vi "SubRotate.vi"(8 "error in (no error)":errorcluster, 10 "input cluster":T1 {"Start X" scale=0.0..1024.0; "End X" scale=0.0..1024.0}, 11 "AVI Path":path) -> (0 "error out":errorcluster)   [LabVIEW 2013]
uses:
  <vilib>/vision/NI_Vision_Development_Module.lvlib
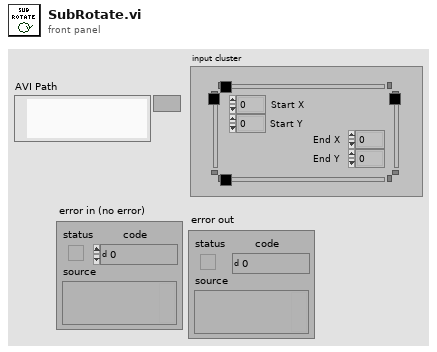
[diagram p1: front panel]
types:
  T1 = typedef "IMAQ Line" = cluster{"Start X":i32, "Start Y":i32, "End X":i32, "End Y":i32}
  T2 = cluster{cluster{i32, i32}, cluster{i32, i32}, cluster{"Start X":i32, "Start Y":i32}, cluster{"End X":i32, "End Y":i32}}
  T3 = typedef "AviRefnum.ctl" = refnum<k1>
  T4 = cluster{"width":u32, "height":u32, "framesPerSecond":u32, "compressionFilter":string, "hasData":bool}
  T5 = typedef "IMAQ Image.ctl" = refnum<image>
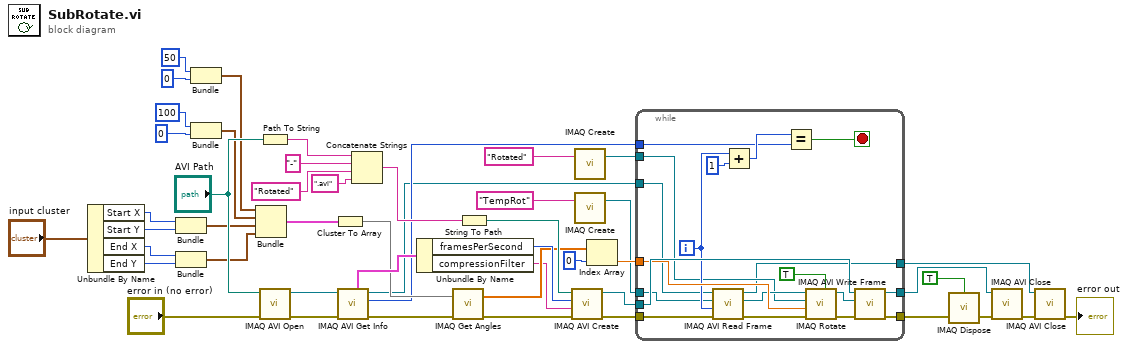
[diagram p0: block diagram]
diagram:
  n1 = Unbundle By Name("input cluster") -> ("Start X"=w30:i32, "Start Y"=w29:i32, "End X"=w28:i32, "End Y"=w27:i32)
  n2 = Bundle("Start X"=w30, "Start Y"=w29) -> (w26:cluster{"Start X":i32, "Start Y":i32})  [unwired: 1 in]
  n3 = Bundle("End X"=w28, "End Y"=w27) -> (w25:cluster{"End X":i32, "End Y":i32})  [unwired: 1 in]
  n4 = Bundle(50, 0) -> (w32:cluster{i32, i32})  [unwired: 1 in]
  n5 = Bundle(100, 0) -> (w31:cluster{i32, i32})  [unwired: 1 in]
  n6 = Bundle(w32, w31, w26, w25) -> (w24:T2)  [unwired: 1 in]
  n7 = Path To String(path="AVI Path") -> (string=w43:string)
  n8 = call "IMAQ AVI Open"("error in (no error)"="error in (no error)", "AVI Path"="AVI Path") -> ("error out"=w48:errorcluster, "Avi Refnum"=w47:T3)  [unwired: 8 in]
  n9 = Cluster To Array(cluster=w24) -> (array=w23:cluster{"End X":i32, "End Y":i32}[])
  n10 = call "IMAQ AVI Get Info"("error in (no error)"=w48, "Avi Refnum"=w47) -> ("error out"=w5:errorcluster, "Number of Frames"=w19:u32, "Avi Refnum (duplicate)"=w4:T3, "Frame Data"=w46:T4)  [unwired: 5 in, 1 out]
  n11 = Concatenate Strings(w43, "-" ("string"), "Rotated" ("string"), ".avi" ("string")) -> (w40:string)
  n12 = Unbundle By Name(w46) -> ("framesPerSecond"=w45:u32, "compressionFilter"=w18:string)
  n13 = call "IMAQ Get Angles"("error in (no error)"=w5, "Points"=w23) -> ("error out"=w17:errorcluster, "Angles (deg)"=w22:sgl[])  [unwired: 3 in, 1 out]
  n14 = String To Path(string=w40) -> (path=w39:path)
  n15 = call "IMAQ AVI Create"("error in (no error)"=w17, "Compression Filter"=w18, "Frames Per Second"=w45, "AVI Path"=w39) -> ("error out"=w7:errorcluster, "Avi Refnum"=w38:T3)  [unwired: 6 in]
  n16 = call "IMAQ Create"("Image Name"="Rotated") -> ("New Image"=w12:T5)  [unwired: 4 in, 1 out]
  n17 = call "IMAQ Create"("Image Name"="TempRot") -> ("New Image"=w14:T5)  [unwired: 4 in, 1 out]
  n18 = Index Array(array=w22, index=0) -> (element=w20:sgl)
  n19 = while {
    tunnel: w38 -> [w67]
    tunnel: [w66] -> w10
    tunnel: [w65] -> w37
    tunnel: w20 -> [w61]
    tunnel: w19 -> [w55]
    tunnel: w14 -> [w53]
    tunnel: w12 -> [w52]
    tunnel: w7 -> [w51]
    tunnel: w4 -> [w50]
    tunnel: [w49] -> w1
    i -> [w58]
    stop <- w54 stop-if-true
    n20 = call "IMAQ AVI Read Frame"("error in (no error)"=w51, "Frame Number"=w58, "Image"=w53, "Avi Refnum"=w50) -> ("error out"=w63:errorcluster, "Image Out"=w60:T5, "Avi Refnum (duplicate)"=w49:T3)  [unwired: 4 in, 1 out]
    n21 = Add(x=w58, y=i8 1) -> (x+y=w56:i32)
    n22 = Equal?(x=w56, y=w55) -> (x = y?=w54:bool)
    n23 = call "IMAQ Rotate"("Maintain Size"=TRUE, "error in (no error)"=w63, "Angle (degrees)"=w61, "Image Dst"=w52, "Image Src"=w60) -> ("error out"=w62:errorcluster, "Image Dst Out"=w59:T5)  [unwired: 5 in]
    n24 = call "IMAQ AVI Write Frame"("error in (no error)"=w62, "Image"=w59, "Avi Refnum"=w67) -> ("error out"=w66:errorcluster, "Avi Refnum (duplicate)"=w65:T3)  [unwired: 7 in]
  }
  n25 = call "IMAQ Dispose"("All Images? (No)"=TRUE, "error in (no error)"=w10) -> ("error out"=w9:errorcluster)  [unwired: 4 in]
  n26 = call "IMAQ AVI Close"("error in (no error)"=w9, "Avi Refnum"=w37) -> ("error out"=w3:errorcluster)  [unwired: 9 in]
  n27 = call "IMAQ AVI Close"("error in (no error)"=w3, "Avi Refnum"=w1) -> ("error out"=→"error out":errorcluster)  [unwired: 9 in]
